vi "injectSample.vi"() -> ()   [LabVIEW 2010]
panel:
  in  "init?":bool=TRUE
  in  "Port Configuration":T1={"baud rate (9600)"=9600, "data bits (8)"=8, "parity (0:none)"=enum."None", "stop bits (10: 1 bit)"=10, "flow control (0:none)"=0, "timeout (10sec)"=10000, "termination char\n(0xA = '\\n' = LF) "=10, "Enable Termination\nChar (T)"=TRUE} {"termination char\n(0xA = '\\n' = LF)" format="%.0x"; "flow control (0:none)" items=["None", "XON/XOFF", "RTS/CTS", "XON/XOFF & RTS/CTS", "DTR/DSR", "XON/XOFF & DTR/DSR"]; "stop bits (10: 1 bit)" items=["1.0"=10, "1.5"=15, "2.0"=20]; "data bits (8)" min=5 max=8 step=1}
  out "error out":errorcluster
  in  "error in":errorcluster
  in  "VISA resource name":refnum<visa-resource-name>="COM10"
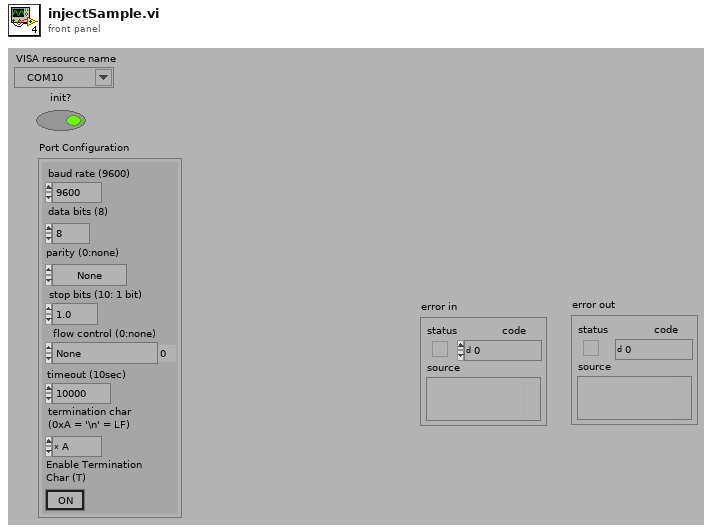
[diagram p1: front panel]
types:
  T1 = cluster{"baud rate (9600)":u32, "data bits (8)":u16, "parity (0:none)":enum16{"None", "Odd", "Even", "Mark", "Space"}, "stop bits (10: 1 bit)":u16, "flow control (0:none)":u16, "timeout (10sec)":u32, "termination char\n(0xA = '\\n' = LF) ":u8, "Enable Termination\nChar (T)":bool}
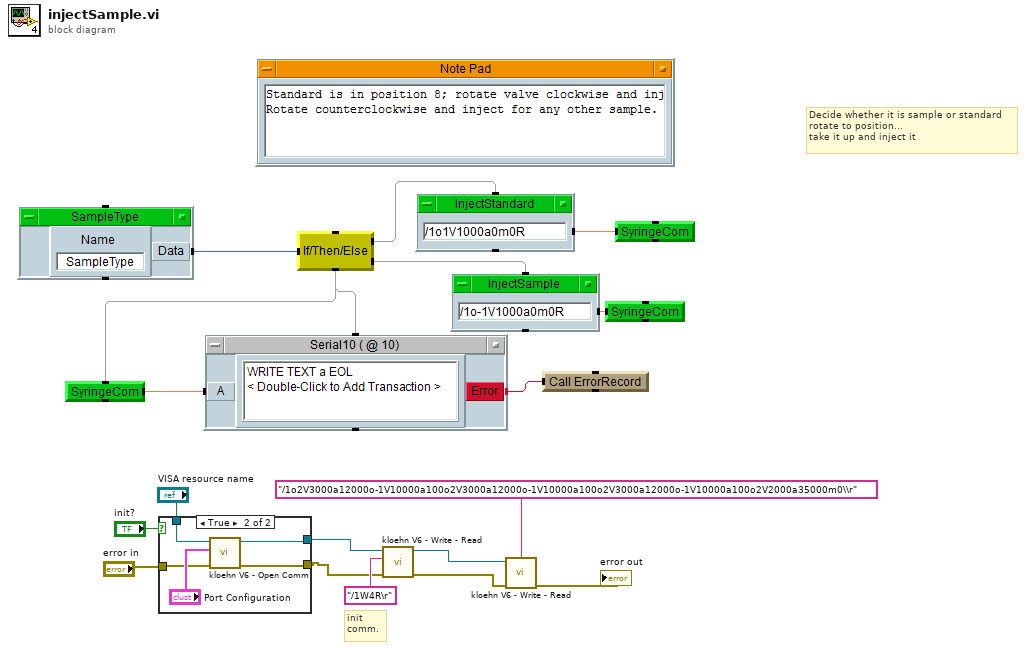
[diagram p0: block diagram]
diagram:
  # "init\ncomm."
  # "Decide whether it is sample or standard\nrotate to position...\ntake it up and inject it"
  n1 = case shown="True" "init?" {
    tunnel: [w11 w14] -> w4
    tunnel: [w12 w13] -> w2
    tunnel: "error in" -> [w12 w16]
    tunnel: "VISA resource name" -> [w11 w15]
    frame False {
    }
    frame True {
      n2 = call "kloehn V6 - Open Comm .vi"("error in"=w16, "Serial Parameters"="Port Configuration", "VISA Ref"=w15) -> ("error out"=w13:errorcluster, "VISA Ref DUP"=w14:refnum<visa-resource-name>)  [unwired: 7 in]
    }
  }
  n3 = call "kloehn V6 - Write - Read.vi"("error in"=w2, "Send String"="/1W4R\r", "VISA Ref"=w4) -> ("error out"=w1:errorcluster, "VISA Ref DUP"=w3:refnum<visa-resource-name>)  [unwired: 4 in, 3 out]
  n4 = call "kloehn V6 - Write - Read.vi"("error in"=w1, "Send String"="/1o2V3000a12000o-1V10000a100o2V3000a12000o-1V10000a100o2V3000a12000o-1V10000a100o2V2000a35000m0\\r", "VISA Ref"=w3) -> ("error out"=→"error out":errorcluster)  [unwired: 4 in, 4 out]
